vi "half addder.vi"(2 "b":bool, 3 "a":bool) -> (0 "carry":bool, 1 "sum":bool)   [LabVIEW 2024]
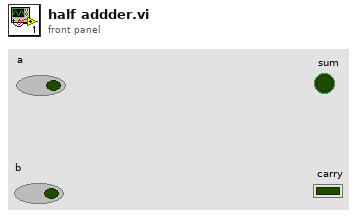
[diagram p1: front panel]
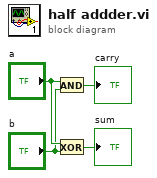
[diagram p0: block diagram]
diagram:
  n1 = And(x="a", y="b") -> (x .and. y?=→"carry":bool)
  n2 = Exclusive Or(1:"b", 2:"a") -> (0:→"sum":bool)
